vi "Set Dev Mode.vi"(6 "cancel refnum":refnum<vi>, 8 "error in (no error)":errorcluster, 9 "firmware revision":string(combo), 10 "dev mode":bool, 11 "VISA resource name":refnum<visa-resource-name>) -> (0 "error out":errorcluster, 2 "bridge error":T1, 3 "VISA resource name out":refnum<visa-resource-name>)   [LabVIEW 2019, in "Andeen-Hagerling 2700A.lvlib"]
doc: "Enables or disables the deviation mode. When enabled, the\ndeviation mode takes capacitance and loss measurements\nvery rapidly and converts them to analog voltages that are\nproportional to the measured capacitance and loss. This is a\nspecial mode of operation that functions as a high-speed\nalternative to the normal bridge mode measurements."
uses:
  Andeen-Hagerling 2700A.lvlib
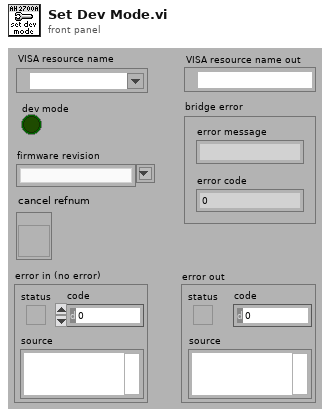
[diagram p1: front panel]
types:
  T1 = cluster{"error message":string, "error code":i32}
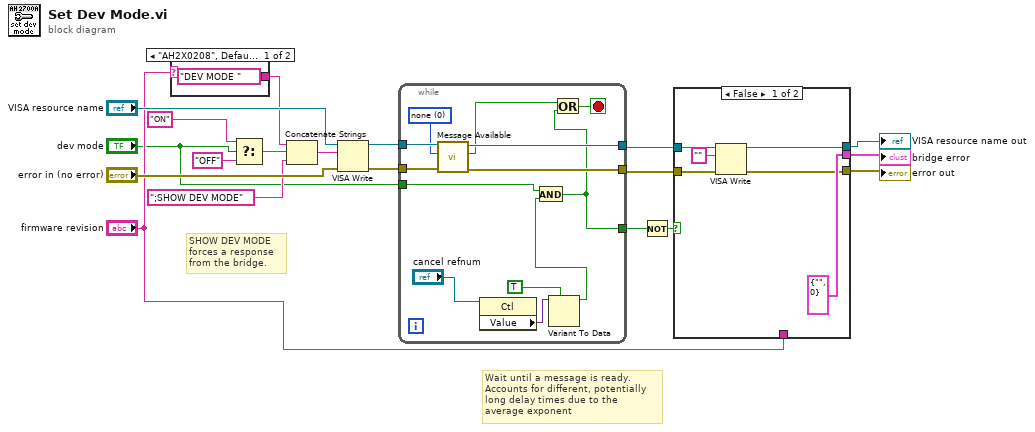
[diagram p0: block diagram]
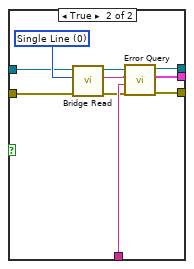
[diagram p2: hidden frame]
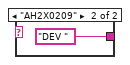
[diagram p3: hidden frame]
diagram:
  # "SHOW DEV MODE\nforces a response\nfrom the bridge."
  # "Wait until a message is ready.\nAccounts for different, potentially\nlong delay times due to the \naverage exponent"
  n1 = case shown="\"AH2X0208\", Default" "firmware revision" {
    tunnel: ["DEV MODE " ("command") "DEV " ("command")] -> w16
    frame "AH2X0208", Default {
    }
    frame "AH2X0209" {
    }
  }
  n2 = Select(t="ON", s="dev mode", f="OFF") -> (s? t:f=w15:string)
  n3 = Concatenate Strings(w16, w15, ";SHOW DEV MODE") -> (w17:string)
  n4 = VISA Write(VISA resource name="VISA resource name", write buffer=w17, error in (no error)="error in (no error)") -> (VISA resource name out=w7:refnum<visa-resource-name>, error out=w6:errorcluster)  [unwired: 1 out]
  n5 = while {
    tunnel: w7 -> [w34]
    tunnel: w6 -> [w33]
    tunnel: [w32] -> w11
    tunnel: [w31] -> w10
    tunnel: [w22] -> w8
    tunnel: "dev mode" -> [w24]
    stop <- w29 stop-if-true
    w30 = u16 0 items=["none", "error check", "multiline read", "infinite"] ("delay")
    n6 = call "Message Available.vi"("error in (no error)"=w33, "delay"=w30, "VISA resource name"=w34) -> ("error out"=w31:errorcluster, "message available"=w28:bool, "VISA resource name out"=w32:refnum<visa-resource-name>)  [unwired: 6 in]
    n7 = property class="Ctl"(reference="cancel refnum") -> ("Value"=w26:variant)  [unwired: 1 in, 2 out]
    n8 = Variant To Data(type=TRUE, Variant=w26) -> (data=w23:bool)  [unwired: 1 in, 1 out]
    n9 = And(x=w24, y=w23) -> (x .and. y?=w22:bool)
    n10 = Or(x=w28, y=w22) -> (x .or. y?=w29:bool)
  }
  n11 = Not(x=w8) -> (.not. x?=w9:bool)
  n12 = case shown="False" w9 {
    tunnel: [w38 w50] -> w5
    tunnel: [w36 w49] -> w3
    tunnel: "firmware revision" -> [_ w48]
    tunnel: [T1 {"error message"="", "error code"=0} ("bridge error") w47] -> w4
    tunnel: w11 -> [w39 w42]
    tunnel: w10 -> [w37 w41]
    frame False {
      n13 = VISA Write(VISA resource name=w39, write buffer="", error in (no error)=w37) -> (VISA resource name out=w38:refnum<visa-resource-name>, error out=w36:errorcluster)  [unwired: 1 out]
    }
    frame True {
      w43 = u16 0 items=["Single Line", "Multi-Line"] ("Multiline")
      n14 = call "Bridge Read.vi"("error in (no error)"=w41, "multiline"=w43, "VISA resource name"=w42) -> ("error out"=w44:errorcluster, "read buffer"=w46:string, "VISA resource name out"=w45:refnum<visa-resource-name>)  [unwired: 6 in]
      n15 = call "Error Query.vi"("error in (no error)"=w44, "firmware revision"=w48, "measurement line"=w46, "VISA resource name"=w45) -> ("error out"=w49:errorcluster, "bridge error"=w47:T1, "VISA resource name out"=w50:refnum<visa-resource-name>)  [unwired: 5 in]
    }
  }
  "VISA resource name out" <- w5
  "error out" <- w3
  "bridge error" <- w4
